vi "List.vi"(8 "error in (no error)":errorcluster, 10 "Key":string, 11 "LUT in":refnum<class "LUT.lvclass">) -> (0 "error out":errorcluster, 1 "Found?":bool, 2 "Values":string[](array[string]), 3 "LUT out":refnum<class "LUT.lvclass">)   [LabVIEW 2016, in "LUT.lvclass"]
uses:
  LUT.lvclass
  LUT.lvclass/LUT.ctl
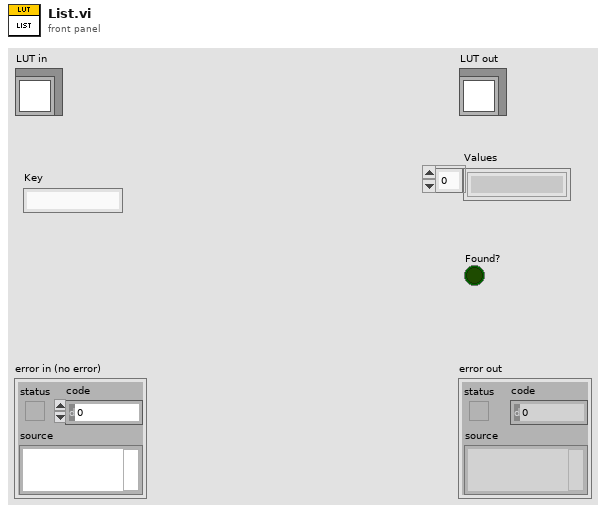
[diagram p1: front panel]
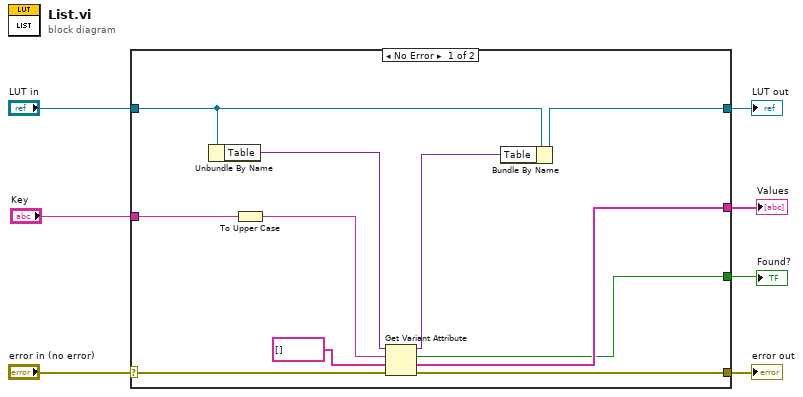
[diagram p0: block diagram]
diagram:
  n1 = case shown="No Error" "error in (no error)" {
    selector: "error in (no error)" -> [w17 w20]
    tunnel: [w16 w20] -> w6
    tunnel: [w13 w19] -> w4
    tunnel: "LUT in" -> [w18 w19]
    tunnel: "Key" -> [w14 _]
    tunnel: [w10 _] -> w2
    tunnel: [w9 _] -> w1
    frame No Error {
      n2 = Unbundle By Name(w18) -> ("Table"=w15:variant)
      n3 = To Upper Case(1:w14) -> (0:w8:string)
      n4 = Get Variant Attribute(Variant=w15, name=w8, default value (empty Variant)=string[] [], error in=w17) -> (duplicate Variant=w12:variant, found=w9:bool, value=w10:string[], error out=w16:errorcluster)
      n5 = Bundle By Name(cluster=w18, "Table"=w12) -> (w13:refnum<class "LUT.lvclass">)
    }
    frame Error {
    }
  }
  "error out" <- w6
  "LUT out" <- w4
  "Values" <- w2
  "Found?" <- w1
